vi "CRYTable to Curve.vi"(11 "Table In":string[][](array[string])) -> (3 "Limit curve":cluster{"Numeric":dbl, "Numeric 2":dbl}[](array[cluster]) {"Numeric 2" format="%.2f"; "Numeric" format="%.2f"})   [LabVIEW 2013]
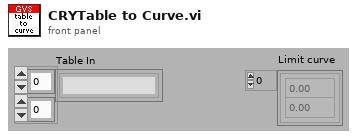
[diagram p1: front panel]
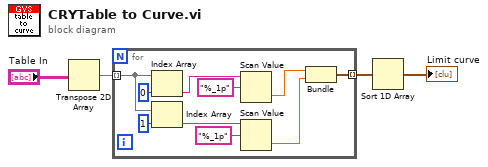
[diagram p0: block diagram]
diagram:
  n1 = Transpose 2D Array(2D array="Table In") -> (transposed array=w4:string[][])
  n2 = for {
    tunnel: w4 -> [w11] mode=indexing
    tunnel: [w14] -> w3 mode=indexing
    n3 = Index Array(array=w11, index=0 ("Index")) -> (element=w10:string)
    n4 = Index Array(array=w11, index=1 ("Index")) -> (element=w9:string)
    n5 = Scan Value(string=w10, format string="%_1p") -> (value=w8:dbl)  [unwired: 1 in, 1 out]
    n6 = Scan Value(string=w9, format string="%_1p") -> (value=w7:dbl)  [unwired: 1 in, 1 out]
    n7 = Bundle(w8, w7) -> (w14:cluster{dbl, dbl})  [unwired: 1 out]
  }
  n8 = Sort 1D Array(array=w3) -> (sorted array=→"Limit curve":cluster{dbl, dbl}[])
